vi "SetupDFUSe.vi"(0 "Error In":errorcluster, 1 "Max Retries":i32=5, 2 "Working Directory":path=path "", 3 "Serial Port":refnum<visa-resource-name>) -> (7 "Error":errorcluster, 10 "Success":bool)   [LabVIEW 2010]
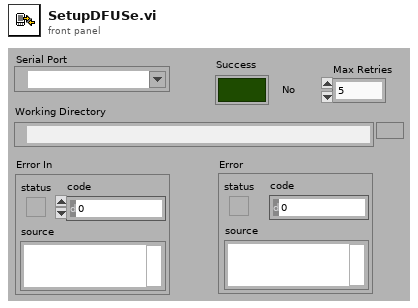
[diagram p1: front panel]
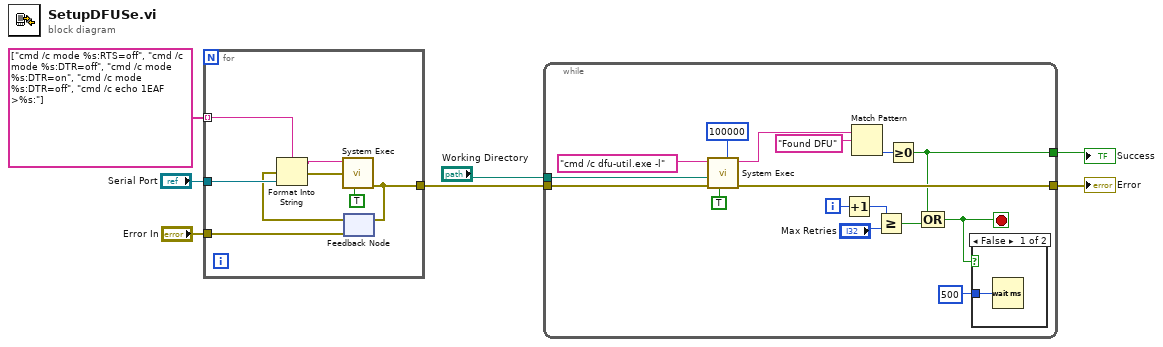
[diagram p0: block diagram]
diagram:
  n1 = for {
    tunnel: "Serial Port" -> [w15]
    tunnel: string[] ["cmd /c mode %s:RTS=off", "cmd /c mode %s:DTR=off", "cmd /c mode %s:DTR=on", "cmd /c mode %s:DTR=off", "cmd /c echo 1EAF >%s:"] -> [w11] mode=indexing
    tunnel: [w10] -> w4
    tunnel: "Error In" -> [w8]
    n2 = feedback #1(w8) -> (w13:errorcluster)
    n3 = Format Into String(format string=w11, error in=w13, w15) -> (resulting string=w14:string, error out=w12:errorcluster)  [unwired: 1 in]
    n4 = call <vilib>:"System Exec.vi"("run minimized? (F)"=TRUE, "error in (no error)"=w12, "command line"=w14) -> ("error out"=w10:errorcluster)  [unwired: 5 in, 3 out]
    n5 = feedback-in #1(w10) -> ()
  }
  n6 = while {
    tunnel: w4 -> [w31]
    tunnel: "Working Directory" -> [w29]
    tunnel: [w28] -> w2
    tunnel: [w19] -> w1
    i -> [w23]
    stop <- w18 stop-if-true
    n7 = call <vilib>:"System Exec.vi"("expected output size  (4096)"=u32 100000, "run minimized? (F)"=TRUE, "error in (no error)"=w31, "working directory"=w29, "command line"="cmd /c dfu-util.exe -l") -> ("error out"=w28:errorcluster, "standard output"=w26:string)  [unwired: 3 in, 2 out]
    n8 = Increment(x=w23) -> (x+1=w21:i32)
    n9 = Match Pattern(string=w26, regular expression="Found DFU") -> (offset past match=w24:i32)  [unwired: 1 in, 3 out]
    n10 = Greater Or Equal?(x=w21, y="Max Retries") -> (x >= y?=w22:bool)
    n11 = Greater Or Equal To 0?(x=w24) -> (x >= 0?=w19:bool)
    n12 = Compound Arithmetic op=OR(w19, w22) -> (w18:bool)
    n13 = case shown="False" w18 {
      tunnel: u32 500 -> [w32 _]
      frame False {
        n14 = Wait (ms)(milliseconds to wait=w32) -> ()  [unwired: 1 out]
      }
      frame True {
      }
    }
  }
  "Error" <- w2
  "Success" <- w1
